vi "sendUnique.vi"(8 "error in (no error)":errorcluster, 9 "Function":i32, 10 "Address":i32, 11 "Mockbus in":refnum<class "Mockbus.lvclass">) -> (0 "error out":errorcluster, 3 "Mockbus out":refnum<class "Mockbus.lvclass">)   [LabVIEW 2015, in "RTMockbus.lvlib" / "Mockbus.lvclass"]
uses:
  Mockbus.lvclass
  Mockbus.lvclass/Mockbus.ctl
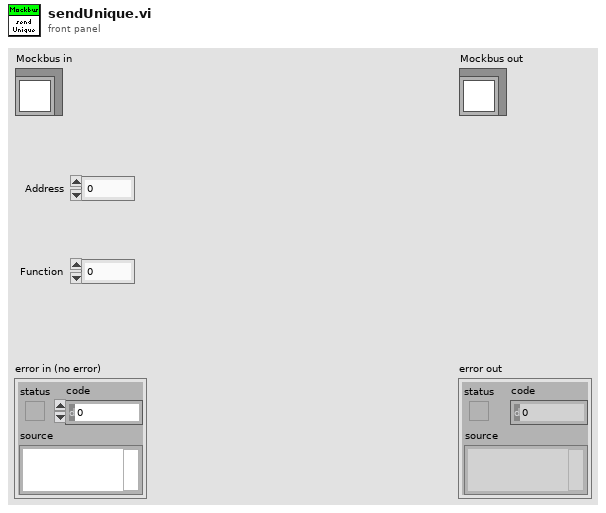
[diagram p1: front panel]
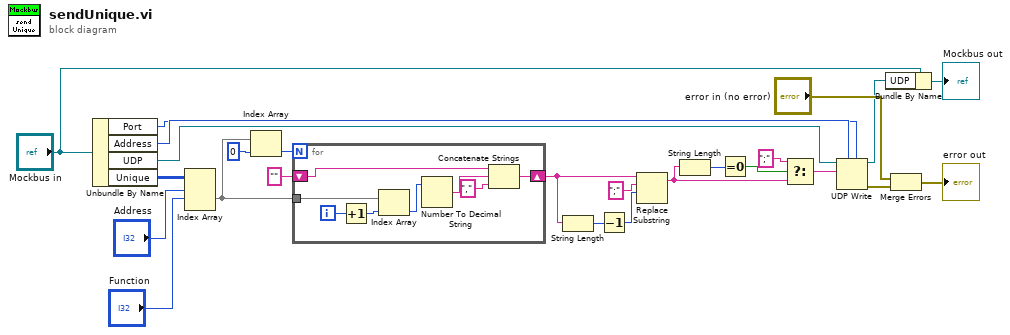
[diagram p0: block diagram]
diagram:
  n1 = Unbundle By Name("Mockbus in") -> ("Port"=w21:u16, "Address"=w22:u32, "UDP"=w23:refnum<k16>, "Unique"=w24:u8[][][])
  n2 = Index Array(array=w24, index (dim 0)="Address", index (dim 1)="Function") -> (element=w11:u8[])  [unwired: 1 in]
  n3 = Index Array(array=w11, index=0) -> (element=w12:u8)
  n4 = for {
    N: w12 -> [_]
    shift-right: [w29] -> w7
    shift-left: "" -> [w28]
    tunnel: w11 -> [w31]
    i -> [w33]
    n5 = Increment(x=w33) -> (x+1=w32:i32)
    n6 = Index Array(array=w31, index=w32) -> (element=w30:u8)
    n7 = Number To Decimal String(number=w30) -> (decimal integer string=w27:string)  [unwired: 1 in]
    n8 = Concatenate Strings(w28, w27, "," ("string")) -> (w29:string)
  }
  n9 = String Length(string=w7) -> (length=w9:i32)
  n10 = Decrement(x=w9) -> (x-1=w10:i32)
  n11 = Replace Substring(3:w10, 4:";" ("substring (\"\")"), 5:w7) -> (1:w4:string)  [unwired: 1 in, 1 out]
  n12 = String Length(string=w4) -> (length=w6:i32)
  n13 = Equal To 0?(x=w6) -> (x = 0?=w5:bool)
  n14 = Select(t=";", s=w5, f=w4) -> (s? t:f=w2:string)
  n15 = UDP Write(address=w22, port or service name=w21, connection ID=w23, data in=w2) -> (error out=w20:errorcluster, 3:w16:refnum<k16>)  [unwired: 2 in]
  n16 = Bundle By Name(cluster="Mockbus in", "UDP"=w16) -> (→"Mockbus out":refnum<class "Mockbus.lvclass">)
  n17 = Merge Errors("error in (no error)", w20) -> (→"error out":errorcluster)
